vi "Edge Plot.vi"(4 "sample rate [Hz]":dbl=11025.0, 5 "time instant\nof pulses":dbl[](array[numeric]) format="%.2e", 7 "Tach signal":dbl[](array[numeric]) format="%.2f") -> (3 "Edge Plot":cluster{"X":dbl[], "Y":dbl[]} {"Y" format="%.2f"; "X" format="%.2f"})   [LabVIEW 2017]
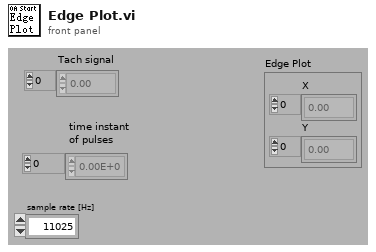
[diagram p1: front panel]
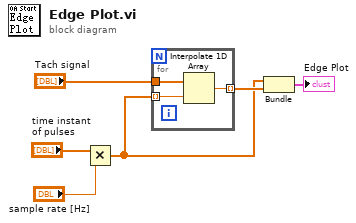
[diagram p0: block diagram]
diagram:
  n1 = Multiply(x="time instant\nof pulses", y="sample rate [Hz]") -> (x*y=w2:dbl[])
  n2 = for {
    tunnel: "Tach signal" -> [w9]
    tunnel: w2 -> [w8] mode=indexing
    tunnel: [w7] -> w5 mode=indexing
    n3 = Interpolate 1D Array(1:w8, 2:w9) -> (0:w7:dbl)
  }
  n4 = Bundle(w2, w5) -> (→"Edge Plot":cluster{dbl[], dbl[]})  [unwired: 1 in]
